vi "Modulation current to field conversion.vi"(10 "Sample holder":T1, 11 "Modulation current (mA)":dbl) -> (3 "Modulation field (G)":dbl)   [LabVIEW 2022 SP3]
uses:
  Datatypes/SampleHolders.ctl
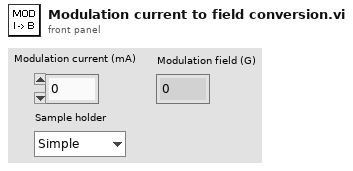
[diagram p1: front panel]
types:
  T1 = typedef "SampleHolders.ctl" = enum16{"Simple", "Carousel", "Chip", "Rotator", "Liquid"}
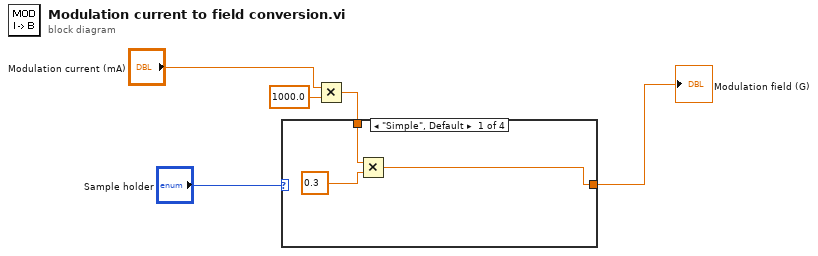
[diagram p0: block diagram]
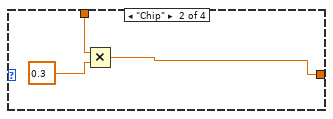
[diagram p2: hidden frame]
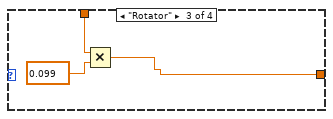
[diagram p3: hidden frame]
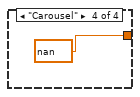
[diagram p4: hidden frame]
diagram:
  n1 = Multiply(x="Modulation current (mA)", y=1000.0) -> (x*y=w4:dbl)
  n2 = case shown="\"Simple\", Default" "Sample holder" {
    tunnel: w4 -> [w7 w10 w13 _]
    tunnel: [w6 w9 w12 nan] -> w3
    frame "Simple", Default {
      n3 = Multiply(x=w7, y=0.3) -> (x*y=w6:dbl)
    }
    frame "Chip" {
      n4 = Multiply(x=w10, y=0.3) -> (x*y=w9:dbl)
    }
    frame "Rotator" {
      n5 = Multiply(x=w13, y=0.099) -> (x*y=w12:dbl)
    }
    frame "Carousel" {
    }
  }
  "Modulation field (G)" <- w3
